vi "UTL_Generar Reporte.vi"(8 "Error in":errorcluster, 10 "Data":dbl[][](array[numeric]), 11 "Results Path":path) -> (0 "Error out":errorcluster, 3 "Tabla de Datos":string[][](array[string]))   [LabVIEW 2019]
uses:
  Variable global de carga.vi
  <vilib>/Utility/file.llb/Read Delimited Spreadsheet (string).vi
  <vilib>/Utility/file.llb/Write Delimited Spreadsheet (string).vi
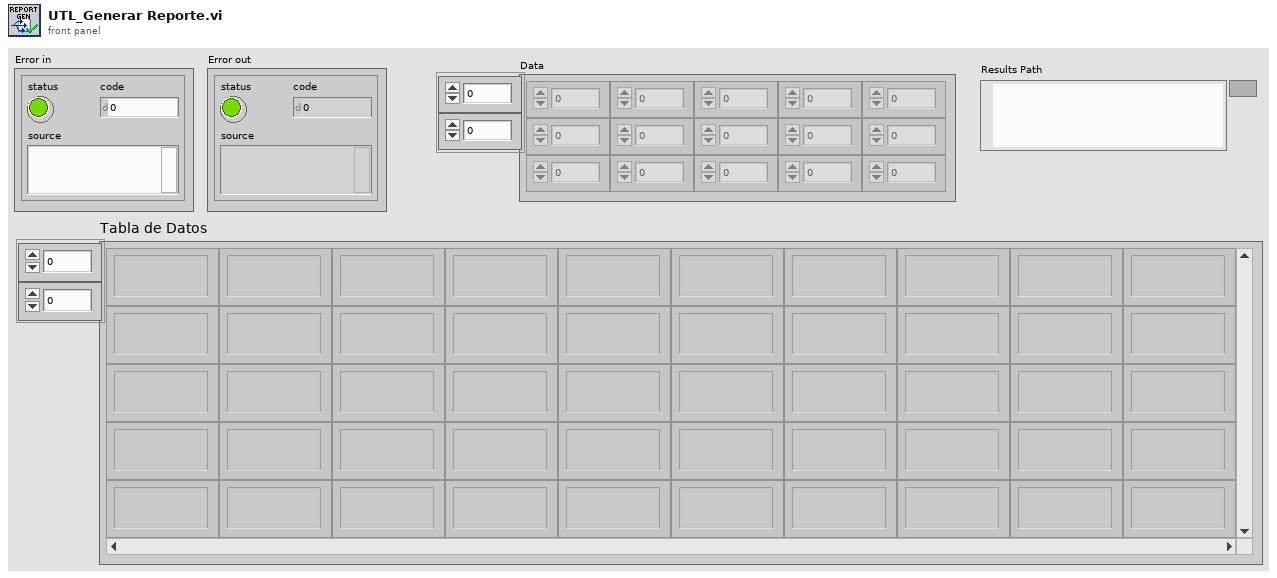
[diagram p1: front panel]
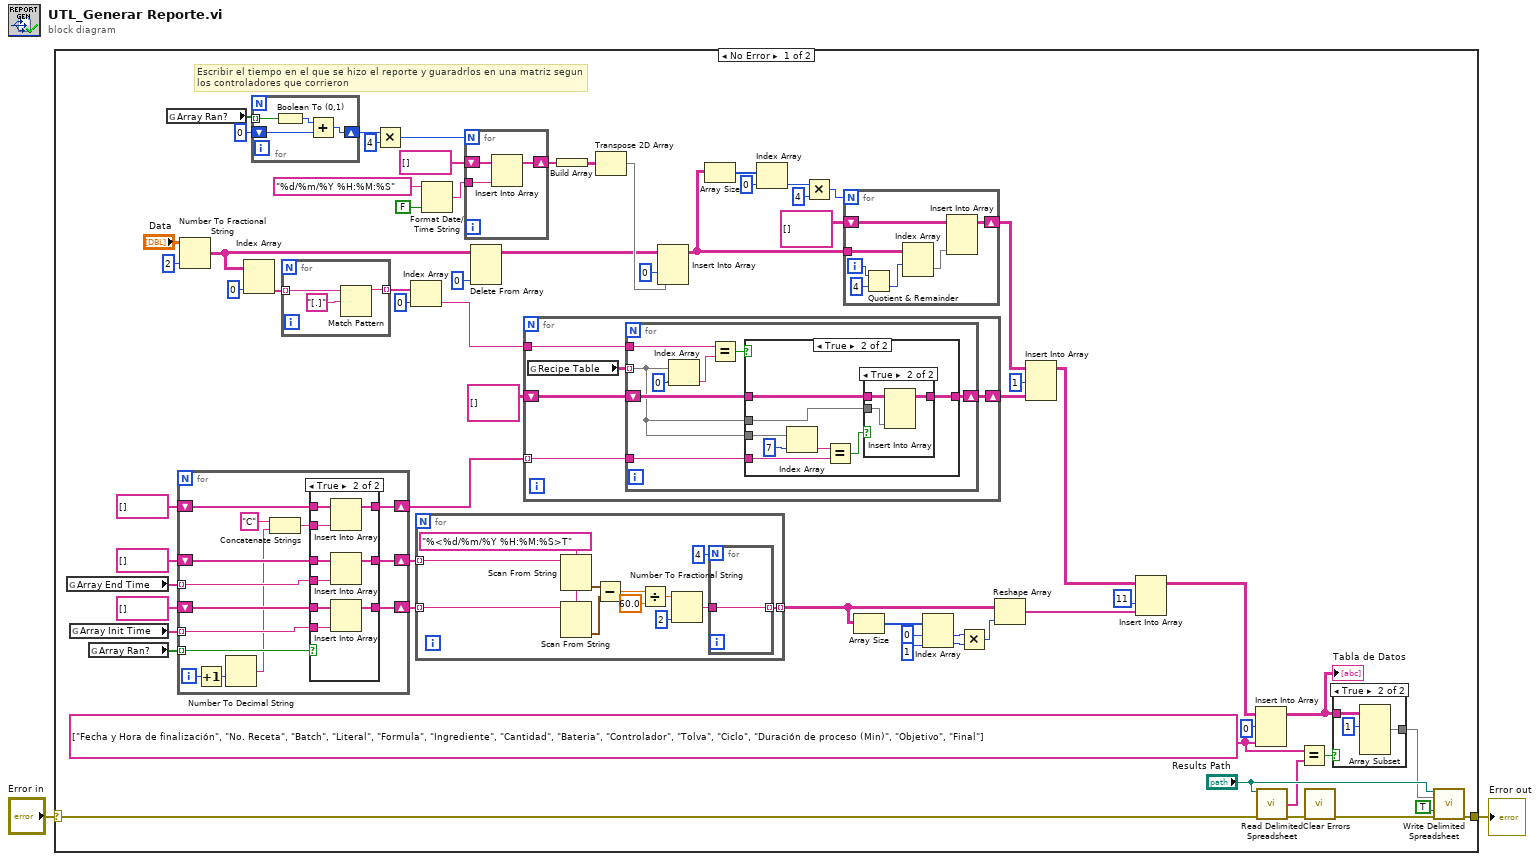
[diagram p0: block diagram]
diagram:
  n1 = case shown="No Error" "Error in" {
    selector: "Error in" -> [w52 w155]
    tunnel: [w62 w155] -> w1
    frame No Error {
      w5 = string[] ["Fecha y Hora de finalización", "No. Receta", "Batch", "Literal", "Formula", "Ingrediente", "Cantidad", "Bateria", "Controlador", "Tolva", "Ciclo", "Duración de proceso (Min)", "Objetivo", "Final"]
      # "Escribir el tiempo en el que se hizo el reporte y guaradrlos en una matriz segun los controladores que corrieron"
      n2 = global read "Variable global de carga.vi" "Array End Time"() -> (w12:string[])
      n3 = global read "Variable global de carga.vi" "Array Init Time"() -> (w13:string[])
      n4 = global read "Variable global de carga.vi" "Array Ran?"() -> (w14:bool[])
      n5 = global read "Variable global de carga.vi" "Array Ran?"() -> (w20:bool[])
      n6 = for {
        tunnel: w14 -> [w95] mode=indexing
        shift-right: [w93] -> w45
        shift-left: string[] [] -> [w94]
        shift-right: [w91] -> w10
        shift-left: string[] [] -> [w92]
        shift-right: [w90] -> w9
        shift-left: string[] [] -> [w89]
        tunnel: w13 -> [w88] mode=indexing
        tunnel: w12 -> [w87] mode=indexing
        i -> [w86]
        n7 = Increment(x=w86) -> (x+1=w85:i32)
        n8 = Number To Decimal String(number=w85) -> (decimal integer string=w84:string)  [unwired: 1 in]
        n9 = Concatenate Strings("C" ("string"), w84) -> (w82:string)
        n10 = case shown="True" w95 {
          tunnel: w94 -> [w98 w107]
          tunnel: [w98 w106] -> w93
          tunnel: w92 -> [w97 w105]
          tunnel: [w97 w104] -> w91
          tunnel: w89 -> [w96 w102]
          tunnel: [w96 w103] -> w90
          tunnel: w88 -> [_ w101]
          tunnel: w87 -> [_ w100]
          tunnel: w82 -> [_ w99]
          frame False {
          }
          frame True {
            n11 = Insert Into Array(array=w107, new element=w99) -> (w106:string[])  [unwired: 1 in]
            n12 = Insert Into Array(array=w105, new element=w100) -> (w104:string[])  [unwired: 1 in]
            n13 = Insert Into Array(array=w102, new element=w101) -> (w103:string[])  [unwired: 1 in]
          }
        }
      }
      n14 = Number To Fractional String(number="Data", precision (6)=i16 2) -> (F-format string=w11:string[][])  [unwired: 2 in]
      n15 = Index Array(array=w11, index (col)=0 ("disabled index (col)")) -> (element=w60:string[])  [unwired: 1 in]
      n16 = for {
        tunnel: w20 -> [w111] mode=indexing
        shift-right: [w108] -> w21
        shift-left: 0 -> [w109]
        n17 = Boolean To (0,1)(Boolean=w111) -> (0, 1=w110:i16)
        n18 = Add(x=w110, y=w109) -> (x+y=w108:i32)
      }
      n19 = for {
        tunnel: w60 -> [w153] mode=indexing
        tunnel: [w152] -> w27 mode=indexing
        n20 = Match Pattern(string=w153, regular expression="[.]") -> (before substring=w152:string)  [unwired: 1 in, 3 out]
      }
      n21 = Multiply(x=w21, y=i16 4) -> (x*y=w19:i32)
      n22 = Index Array(array=w27, index=0) -> (element=w58:string)
      n23 = for {
        tunnel: w10 -> [w70] mode=indexing
        tunnel: w9 -> [w71] mode=indexing
        tunnel: [w69] -> w8 mode=indexing
        w72 = "%<%d/%m/%Y %H:%M:%S>T" ("format string")
        n24 = Scan From String(format string=w72, input string=w70) -> (output 1=w76:timestamp)  [unwired: 3 in, 3 out]
        n25 = Scan From String(format string=w72, input string=w71) -> (output 1=w77:timestamp)  [unwired: 3 in, 3 out]
        n26 = Subtract(x=w76, y=w77) -> (x-y=w79:dbl)
        n27 = Divide(x=w79, y=60.0) -> (x/y=w78:dbl)
        n28 = Number To Fractional String(number=w78, precision (6)=i16 2) -> (F-format string=w80:string)  [unwired: 2 in]
        n29 = for {
          N: 4 -> [_]
          tunnel: w80 -> [w81]
          tunnel: [w81] -> w69 mode=indexing
        }
      }
      n30 = Format Date/Time String(time format string (%c)="%d/%m/%Y %H:%M:%S", UTC format=FALSE) -> (date/time string=w46:string)  [unwired: 1 in]
      n31 = for {
        N: w19 -> [_]
        tunnel: w46 -> [w147]
        shift-right: [w145] -> w47
        shift-left: string[] [] -> [w146]
        n32 = Insert Into Array(array=w146, new element=w147) -> (w145:string[])  [unwired: 1 in]
      }
      n33 = Delete From Array(array=w11, index (col)=0 ("disabled index (col)")) -> (array with subset deleted=w26:string[][])  [unwired: 2 in, 1 out]
      n34 = for {
        tunnel: w58 -> [w123]
        tunnel: w45 -> [w122] mode=indexing
        shift-right: [w120] -> w56
        shift-left: string[][] [] -> [w121]
        n35 = global read "Variable global de carga.vi" "Recipe Table"() -> (w119:string[][])
        n36 = for {
          tunnel: w119 -> [w126] mode=indexing
          tunnel: w123 -> [w125]
          tunnel: w122 -> [w129]
          shift-right: [w127] -> w120
          shift-left: w121 -> [w128]
          n37 = Index Array(array=w126, index=0) -> (element=w124:string)
          n38 = Equal?(x=w125, y=w124) -> (x = y?=w130:bool)
          n39 = case shown="True" w130 {
            tunnel: w126 -> [_ w140]
            tunnel: w129 -> [_ w137]
            tunnel: [w132 w134] -> w127
            tunnel: w128 -> [w132 w135]
            tunnel: w126 -> [_ w133]
            frame False {
            }
            frame True {
              n40 = Index Array(array=w140, index=7) -> (element=w138:string)
              n41 = Equal?(x=w138, y=w137) -> (x = y?=w136:bool)
              n42 = case shown="True" w136 {
                tunnel: w135 -> [w141 w144]
                tunnel: [w141 w143] -> w134
                tunnel: w133 -> [_ w142]
                frame False {
                }
                frame True {
                  n43 = Insert Into Array(array=w144, new element=w142) -> (w143:string[][])  [unwired: 2 in]
                }
              }
            }
          }
        }
      }
      n44 = Build Array(w47) -> (w65:string[][])
      n45 = Transpose 2D Array(2D array=w65) -> (transposed array=w64:string[][])
      n46 = Insert Into Array(array=w26, index (col)=0 ("disabled index (col)"), new element=w64) -> (w41:string[][])  [unwired: 1 in]
      n47 = Array Size(array=w41) -> (size(s)=w40:i32[])
      n48 = Index Array(array=w40, index=0) -> (element=w38:i32)
      n49 = Multiply(x=w38, y=i16 4) -> (x*y=w37:i32)
      n50 = for {
        N: w37 -> [_]
        tunnel: w41 -> [w115]
        shift-right: [w113] -> w36
        shift-left: string[][] [] -> [w114]
        i -> [w118]
        n51 = Quotient & Remainder(x=w118, y=4) -> (floor(x/y)=w116:i32)  [unwired: 1 out]
        n52 = Index Array(array=w115, index (row)=w116) -> (element=w112:string[])  [unwired: 1 in]
        n53 = Insert Into Array(array=w114, new element=w112) -> (w113:string[][])  [unwired: 2 in]
      }
      n54 = Array Size(array=w8) -> (size(s)=w35:i32[])
      n55 = Index Array(array=w35, index #1=0 ("index"), index #2=1 ("index")) -> (element #1=w32:i32, element #2=w31:i32)
      n56 = Multiply(x=w32, y=w31) -> (x*y=w30:i32)
      n57 = Reshape Array(w8, w30) -> (w29:string[])
      n58 = Insert Into Array(array=w36, index (col)=1, new element=w56) -> (w7:string[][])  [unwired: 1 in]
      n59 = Insert Into Array(array=w7, index (col)=11 ("disabled index (col)"), new element=w29) -> (w54:string[][])  [unwired: 1 in]
      n60 = Insert Into Array(array=w54, index (row)=0, new element=w5) -> (w28:string[][])  [unwired: 1 in]
      "Tabla de Datos" <- w28
      n61 = call-poly <vilib>:"Read Delimited Spreadsheet.vi"("file path (dialog if empty)"="Results Path", "error in (no error)"=w52) -> ("first row"=w4:string[], "error out"=w49:errorcluster)  [unwired: 8 in, 4 out]
      n62 = Equal?(x=w5, y=w4) -> (x = y?=w61:bool)
      n63 = call <vilib>:"Clear Errors.vi"("error in (no error)"=w49) -> ("error out"=w3:errorcluster)  [unwired: 5 in, 1 out]
      n64 = case shown="True" w61 {
        tunnel: w28 -> [w148 w151]
        tunnel: [w148 w150] -> w24
        frame False {
        }
        frame True {
          n65 = Array Subset(array=w151, index (row)=1 ("index")) -> (w150:string[][])  [unwired: 3 in]
        }
      }
      n66 = call-poly <vilib>:"Write Delimited Spreadsheet.vi"("file path (dialog if empty)"="Results Path", "2D data"=w24, "append to file? (new file:F)"=TRUE, "error in (no error)"=w3) -> ("error out"=w62:errorcluster)  [unwired: 10 in, 1 out]
    }
    frame Error {
    }
  }
  "Error out" <- w1
